vi "get_IMAQ_refs.vi"(8 "error in (no error)":errorcluster, 11 "ImageCollection in":refnum<class "ImageCollection.lvclass">) -> (0 "error out":errorcluster, 2 "IMAQ refs":T1[](array[typedef]), 3 "ImageCollection out":refnum<class "ImageCollection.lvclass">)   [LabVIEW 2010, in "ImageCollection.lvclass"]
uses:
  ImageCollection.lvclass
  <vilib>/vision/Image Controls.llb/IMAQ Image.ctl
  Image/Image/Image.lvclass
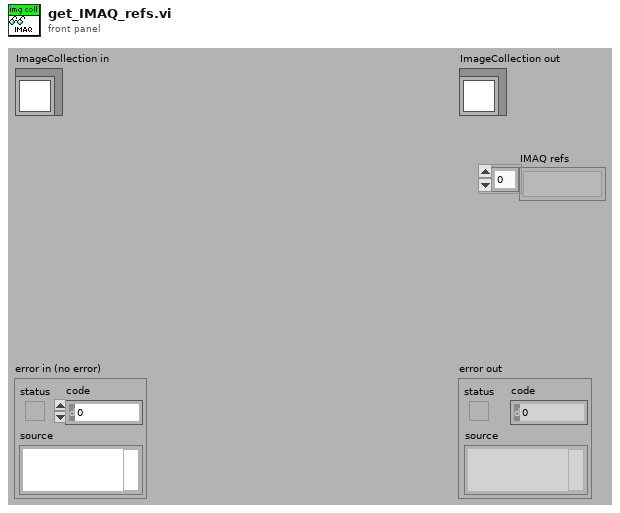
[diagram p1: front panel]
types:
  T1 = typedef "IMAQ Image.ctl" = refnum<image>
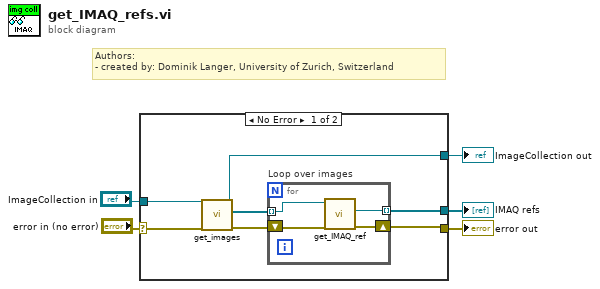
[diagram p0: block diagram]
diagram:
  # "Authors: \n- created by: Dominik Langer, University of Zurich, Switzerland"
  n1 = case shown="No Error" "error in (no error)" {
    selector: "error in (no error)" -> [w12 w18]
    tunnel: [w7 w18] -> w4
    tunnel: [w10 w17] -> w2
    tunnel: "ImageCollection in" -> [w11 w17]
    tunnel: [w6 _] -> w1
    frame No Error {
      n2 = call-dynamic "get_images.vi"("error in (no error)"=w12, "ImageCollection.lvclass in"=w11) -> ("error out"=w9:errorcluster, "images"=w8:refnum<class "Image.lvclass">[], "ImageCollection.lvclass out"=w10:refnum<class "ImageCollection.lvclass">)  [unwired: 7 out]
      n3 = for "Loop over images" {
        tunnel: w8 -> [w15] mode=indexing
        tunnel: [w14] -> w6 mode=indexing
        shift-right: [w13] -> w7
        shift-left: w9 -> [w16]
        n4 = call-dynamic "get_IMAQ_ref.vi"("error in (no error)"=w16, "Image.lvclass in"=w15) -> ("error out"=w13:errorcluster, "Image"=w14:T1)  [unwired: 8 out]
      }
    }
    frame Error {
    }
  }
  "error out" <- w4
  "ImageCollection out" <- w2
  "IMAQ refs" <- w1
